vi "Find Start.vi"(8 "error in (no error)":errorcluster, 11 "2DArrayManager in":refnum<class "2DArrayManager.lvclass">) -> (0 "error out":errorcluster, 3 "2DArrayManager out":refnum<class "2DArrayManager.lvclass">)   [LabVIEW 2020, in "OOPanel.lvlib" / "2DArrayManager.lvclass"]
uses:
  2DArrayManager.lvclass
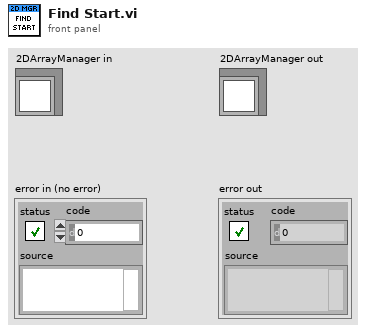
[diagram p1: front panel]
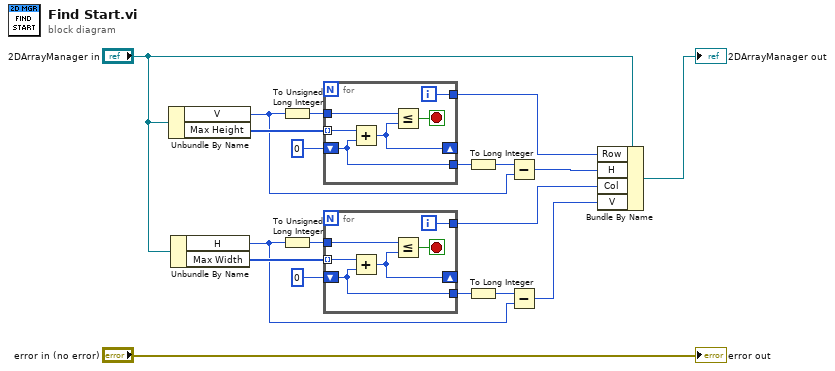
[diagram p0: block diagram]
diagram:
  n1 = Unbundle By Name("2DArrayManager in") -> ("V"=w9:i32, "Max Height"=w13:i32[])
  n2 = Unbundle By Name("2DArrayManager in") -> ("H"=w3:i32, "Max Width"=w4:i32[])
  n3 = To Unsigned Long Integer(number=w9) -> (unsigned 32bit integer=w15:u32)
  n4 = To Unsigned Long Integer(number=w3) -> (unsigned 32bit integer=w6:u32)
  n5 = for {
    tunnel: w15 -> [w25]
    tunnel: w13 -> [w23] mode=indexing
    shift-right: [w22] -> _
    shift-left: u32 0 -> [w20]
    tunnel: [w21] -> w12
    tunnel: [w20] -> w16
    i -> [w21]
    stop <- w24 stop-if-true
    n6 = Add(x=w23, y=w20) -> (x+y=w22:u32)
    n7 = Less Or Equal?(x=w25, y=w22) -> (x <= y?=w24:bool)
  }
  n8 = for {
    tunnel: w6 -> [w31]
    tunnel: w4 -> [w29] mode=indexing
    shift-right: [w28] -> _
    shift-left: u32 0 -> [w26]
    tunnel: [w27] -> w2
    tunnel: [w26] -> w5
    i -> [w27]
    stop <- w30 stop-if-true
    n9 = Add(x=w29, y=w26) -> (x+y=w28:u32)
    n10 = Less Or Equal?(x=w31, y=w28) -> (x <= y?=w30:bool)
  }
  n11 = To Long Integer(number=w16) -> (32bit integer=w11:i32)
  n12 = To Long Integer(number=w5) -> (32bit integer=w8:i32)
  n13 = Subtract(x=w11, y=w9) -> (x-y=w10:i32)
  n14 = Subtract(x=w8, y=w3) -> (x-y=w1:i32)
  n15 = Bundle By Name(cluster="2DArrayManager in", "Row"=w12, "H"=w10, "Col"=w2, "V"=w1) -> (→"2DArrayManager out":refnum<class "2DArrayManager.lvclass">)
  "error out" <- "error in (no error)"
